vi "Parse Dual Remote Terminal.vi"(8 "error in (no error)":errorcluster, 11 "Dual RT XML Node":refnum<k20>) -> (0 "error out":errorcluster, 3 "Dual RT":refnum<class "Remote Terminal.lvclass">[](array[class]))   [LabVIEW 2016]
uses:
  Remote Terminal/Remote Terminal.lvclass
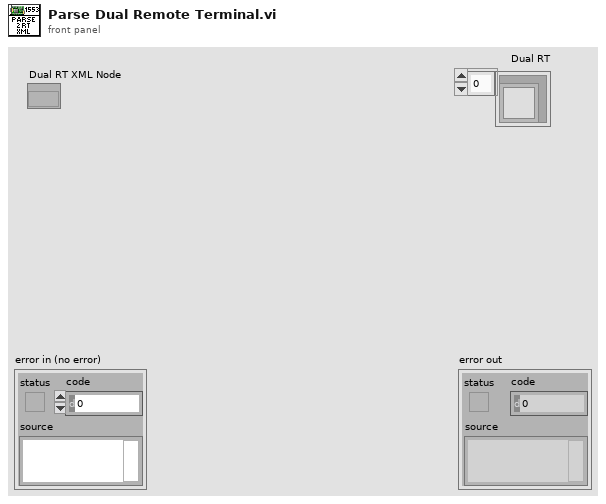
[diagram p1: front panel]
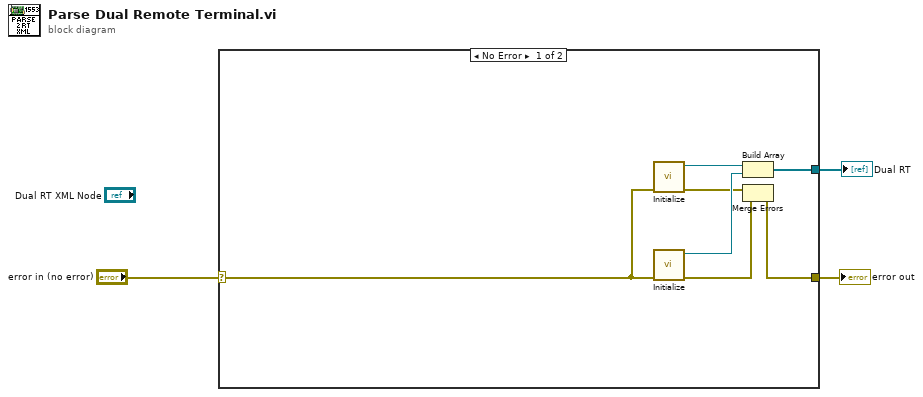
[diagram p0: block diagram]
diagram:
  n1 = case shown="No Error" "error in (no error)" {
    selector: "error in (no error)" -> [w6 w11]
    tunnel: [w5 w11] -> w2
    tunnel: [w4 _] -> w1
    frame No Error {
      n2 = call "Initialize.vi"("error in (no error)"=w6) -> ("error out"=w8:errorcluster, "Remote Terminal out"=w10:refnum<class "Remote Terminal.lvclass">)  [unwired: 9 in]
      n3 = call "Initialize.vi"("error in (no error)"=w6) -> ("error out"=w7:errorcluster, "Remote Terminal out"=w9:refnum<class "Remote Terminal.lvclass">)  [unwired: 9 in]
      n4 = Build Array(w10, w9) -> (w4:refnum<class "Remote Terminal.lvclass">[])
      n5 = Merge Errors(w8, w7) -> (w5:errorcluster)
    }
    frame Error {
    }
  }
  "error out" <- w2
  "Dual RT" <- w1
